vi "Set Up Dialog - Colorimeter.vi"() -> ()   [LabVIEW 2012]
panel:
  in  "Done":bool
  # "iWorx - Colorimeter - Set Up"
  # "Calibration Instructions"
  # "1. Connect the IX-MYDAQ Sensor Adaptor to the NI myDAQ edge connector.\n\n2. Connect the CTSN-100 Colorimeter & Turbidity sensor to the IX-MYDAQ.\n\n3. Connect the NI myDAQ to your computer using a USB cable.\n\n4. Set the sensor to Colorimeter mode. The sensor will only accept micro cuvette's.\n\n5. Prepare a clean cuvette with distilled water. The voltage should be 2.5V for all colors.\n\n6. Prepare another cuvette with black solution to block out all light. The output voltage should be 0V for all colors."
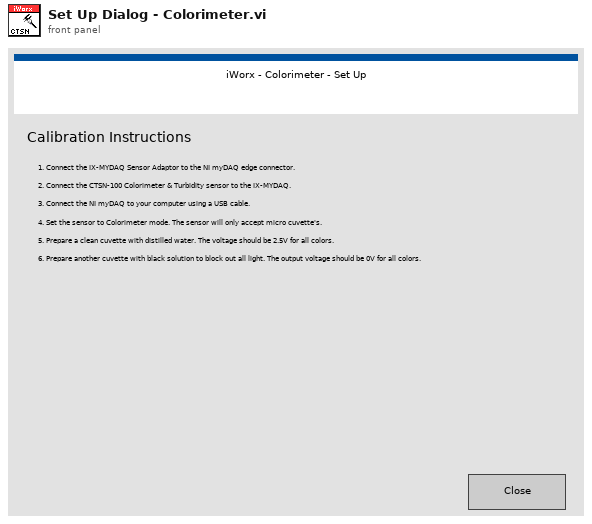
[diagram p1: front panel]
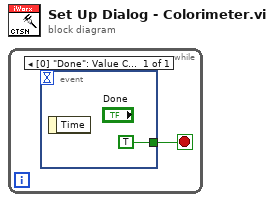
[diagram p0: block diagram]
diagram:
  n1 = while {
    stop <- w1 stop-if-true
    n2 = event shown="[0] \"Done\": Value Change;  Panel Close" {
      selector: _ -> [_]
      dyn-events: _ -> [_]
      timeout: _ -> [_]
      tunnel: [TRUE] -> w1
      event "Done": Value Change; Panel Close {
        n3 = event-data() -> ()  [unwired: 1 in, 1 out]
      }
    }
  }
